vi "Get Setpoint.vi"(1 "GPIB Adress":i16) -> (0 "Temperature":dbl format="%.2f")   [LabVIEW 2015]
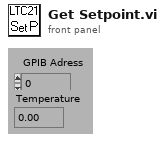
[diagram p1: front panel]
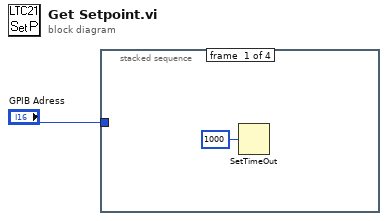
[diagram p0: block diagram]
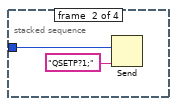
[diagram p2: hidden frame]
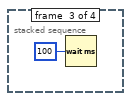
[diagram p3: hidden frame]
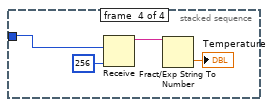
[diagram p4: hidden frame]
diagram:
  n1 = stacked-sequence {
    tunnel: "GPIB Adress" -> [_ w4 _ w9]
    frame #0 {
      n2 = SetTimeOut(1:1000 ("new timeout (10000)")) -> ()  [unwired: 1 out]
    }
    frame #1 {
      n3 = Send(2:w4, 5:"QSETP?1;" ("data string")) -> ()  [unwired: 3 in, 3 out]
    }
    frame #2 {
      n4 = Wait (ms)(milliseconds to wait=u32 100) -> ()  [unwired: 1 out]
    }
    frame #3 {
      n5 = Receive(6:256 ("count"), 8:w9) -> (3:w8:string)  [unwired: 3 in, 3 out]
      n6 = Fract/Exp String To Number(string=w8) -> (number=→"Temperature":dbl)  [unwired: 3 in, 1 out]
    }
  }
